vi "Do.vi"(8 "error in (no error)":errorcluster, 10 "Actor in":refnum<class "Actor.lvclass">, 11 "Unregister Next Button Visibility Msg":refnum<class "Unregister Next Button Visibility Msg.lvclass">) -> (0 "error out":errorcluster, 2 "Actor out":refnum<class "Actor.lvclass">)   [LabVIEW 2013, in "Project Model.lvlib" / "Unregister Next Button Visibility Msg.lvclass"]
doc: "This VI delivers the message to the actor by calling the appropriate method(s) on the actor."
uses:
  Unregister Next Button Visibility Msg.lvclass
  <vilib>/ActorFramework/Actor/Actor.lvclass
  Project Model/Project Model.lvclass
  <vilib>/ActorFrameworkMVC/View Observer/Unregistration Message/Unregistration Message.lvclass/Unregistration Message.ctl
  <vilib>/ActorFramework/Message Enqueuer/Message Enqueuer.lvclass
  <vilib>/ActorFrameworkMVC/View Observer/Unregistration Message/Unregistration Message.lvclass
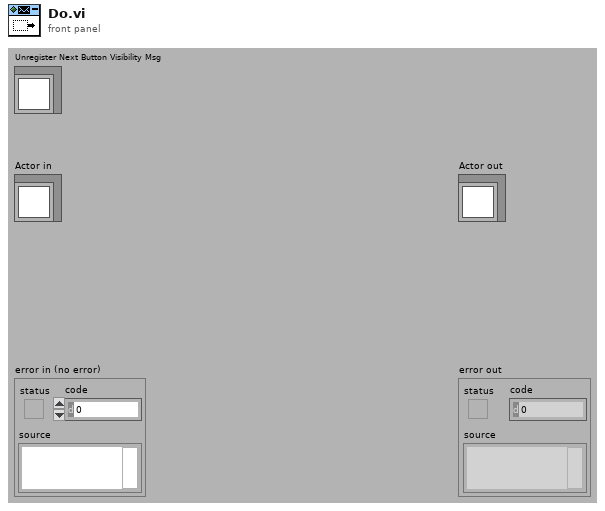
[diagram p1: front panel]
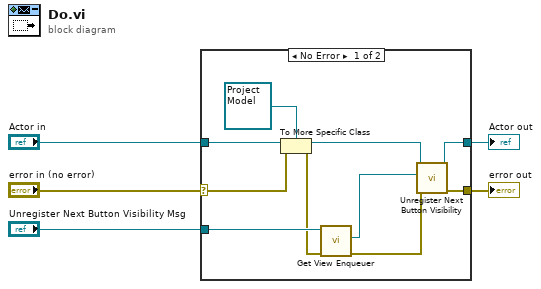
[diagram p0: block diagram]
diagram:
  n1 = case shown="No Error" "error in (no error)" {
    selector: "error in (no error)" -> [w8 w17]
    tunnel: "Unregister Next Button Visibility Msg" -> [w15 _]
    tunnel: "Actor in" -> [w14 w16]
    tunnel: [w11 w16] -> w1
    tunnel: [w9 w17] -> w3
    frame No Error {
      n2 = To More Specific Class(target class=refnum<class "Project Model.lvclass"> refnum ("Model Actor.lvlib:Model Actor.lvclass"), reference=w14, error in=w8) -> (specific class reference=w12:refnum<class "Project Model.lvclass">, error out=w7:errorcluster)
      n3 = call <vilib>:"Get View Enqueuer.vi"("error in (no error)"=w7, "Unregistration Message in"=w15) -> ("error out"=w6:errorcluster, "View Enqueuer"=w10:refnum<class "Message Enqueuer.lvclass">)  [unwired: 7 in, 1 out]
      n4 = call "Unregister Next Button Visibility.vi"("error in (no error)"=w6, "View Enqueuer"=w10, "Project Model in"=w12) -> ("error out"=w9:errorcluster, "Project Model out"=w11:refnum<class "Project Model.lvclass">)  [unwired: 7 in]
    }
    frame Error {
    }
  }
  "error out" <- w3
  "Actor out" <- w1
